vi "TwoBallAutoGlobals.vi"() -> ()   [LabVIEW 2015]
panel:
  out "GyroValue":dbl
  in  "Enum":T1(ring)
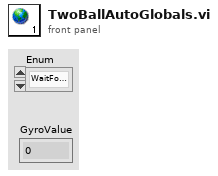
[diagram p1: front panel]
types:
  T1 = enum16{"WaitForInput", "StartIntake", "LowerArm", "IntakeBall", "TurnAndZeroEnc", "DriveForward", "RecordGyro", "TargetAndLoad", "Shoot", "TurnBack", "BackUpAndIntake", "IntakeBall2", "DriveForward2", "TargetAndLoad2", "Shoot2", "End"}
diagram:
